vi "make_random.vi"() -> (1 "key":string)   [LabVIEW 2017, in "Lib_code.lvlib"]
uses:
  Lib_code.lvlib
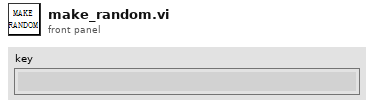
[diagram p1: front panel]
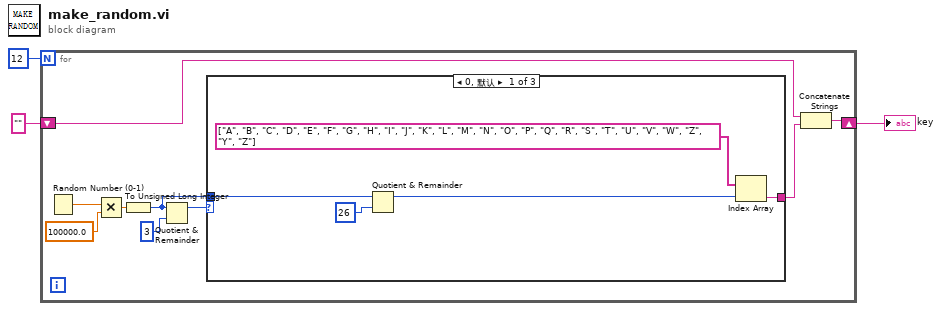
[diagram p0: block diagram]
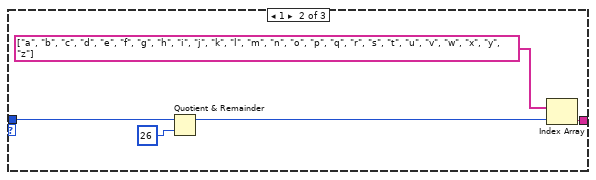
[diagram p2: hidden frame]
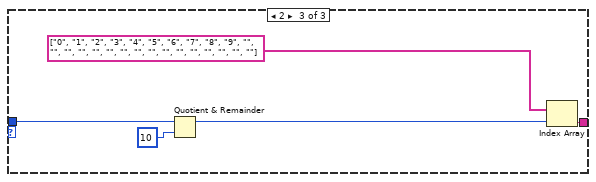
[diagram p3: hidden frame]
diagram:
  n1 = for {
    N: 12 -> [_]
    shift-right: [w12] -> w1
    shift-left: "" -> [w11]
    n2 = Random Number (0-1)() -> (number: 0 to 1=w9:dbl)
    n3 = Multiply(x=w9, y=100000.0) -> (x*y=w5:dbl)
    n4 = To Unsigned Long Integer(number=w5) -> (unsigned 32bit integer=w4:u32)
    n5 = Quotient & Remainder(x=w4, y=u32 3) -> (x-y*floor(x/y)=w6:u32)  [unwired: 1 out]
    n6 = case shown="0, 默认" w6 {
      tunnel: w4 -> [w16 w22 w27]
      tunnel: [w13 w19 w24] -> w10
      frame 0, Default {
        n7 = Quotient & Remainder(x=w16, y=u32 26) -> (x-y*floor(x/y)=w14:u32)  [unwired: 1 out]
        n8 = Index Array(array=string[] ["A", "B", "C", "D", "E", "F", "G", "H", "I", "J", "K", "L", "M", "N", "O", "P", "Q", "R", "S", "T", "U", "V", "W", "Z", "Y", "Z"], index=w14) -> (element=w13:string)
      }
      frame 1 {
        n9 = Quotient & Remainder(x=w22, y=u32 26) -> (x-y*floor(x/y)=w20:u32)  [unwired: 1 out]
        n10 = Index Array(array=string[] ["a", "b", "c", "d", "e", "f", "g", "h", "i", "j", "k", "l", "m", "n", "o", "p", "q", "r", "s", "t", "u", "v", "w", "x", "y", "z"], index=w20) -> (element=w19:string)
      }
      frame 2 {
        n11 = Quotient & Remainder(x=w27, y=u32 10) -> (x-y*floor(x/y)=w25:u32)  [unwired: 1 out]
        n12 = Index Array(array=string[] ["0", "1", "2", "3", "4", "5", "6", "7", "8", "9", "", "", "", "", "", "", "", "", "", "", "", "", "", "", "", ""], index=w25) -> (element=w24:string)
      }
    }
    n13 = Concatenate Strings(w11, w10) -> (w12:string)
  }
  "key" <- w1
